vi "Flat Top Window.vi"   [LabVIEW 2014, in "NI_AALPro.lvlib"]
doc: "Applies a flat top window to the input sequence <B>X</B>. Wire data to the <B>X</B> input to determine the polymorphic instance to use or manually select the instance."
uses:
  NI_AALPro.lvlib
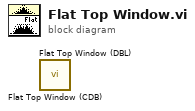
[diagram p0: block diagram]
diagram:
  n1 = call "Flat Top Window (CDB).vi"() -> ()  [unwired: 1 in, 2 out]
  n2 = call "Flat Top Window (DBL).vi"() -> ()  [unwired: 1 in, 2 out]
